vi "lib Read Only 699 Config File.vi"(7 "Mission":string, 8 "error in (no error)":errorcluster, 11 "mission folders in":T1) -> (0 "error out":errorcluster, 3 "mission folders out":T1)   [LabVIEW 2014]
uses:
  lib cluster 699 Config.ctl
  <vilib>/Utility/sysdir.llb/System Directory Type.ctl
  <vilib>/Utility/config.llb/Read Key (String).vi
  <vilib>/Utility/config.llb/NI_LVConfig.lvlib
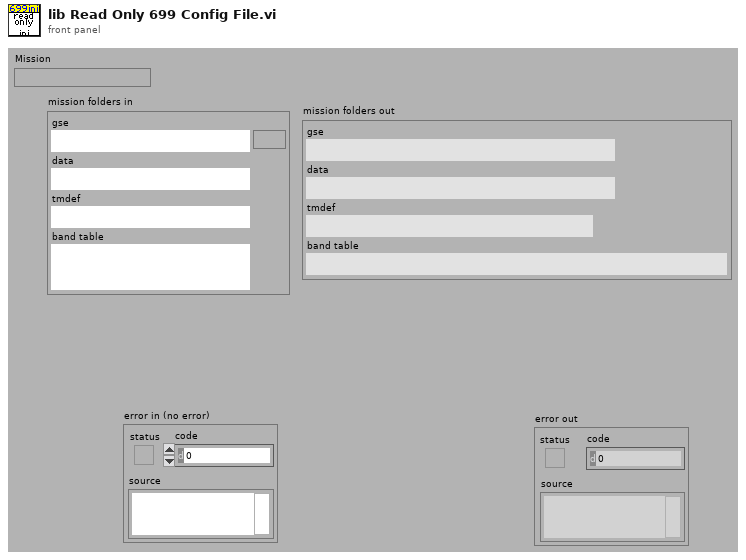
[diagram p1: front panel]
types:
  T1 = typedef "lib cluster 699 Config.ctl" = cluster{"gse":path, "data":path, "tmdef":path, "band table":path}
  T2 = typedef "System Directory Type.ctl" = i32
  T3 = typedef "NI_LVConfig.lvlib/Config Data RefNum.ctl" = refnum<k1>
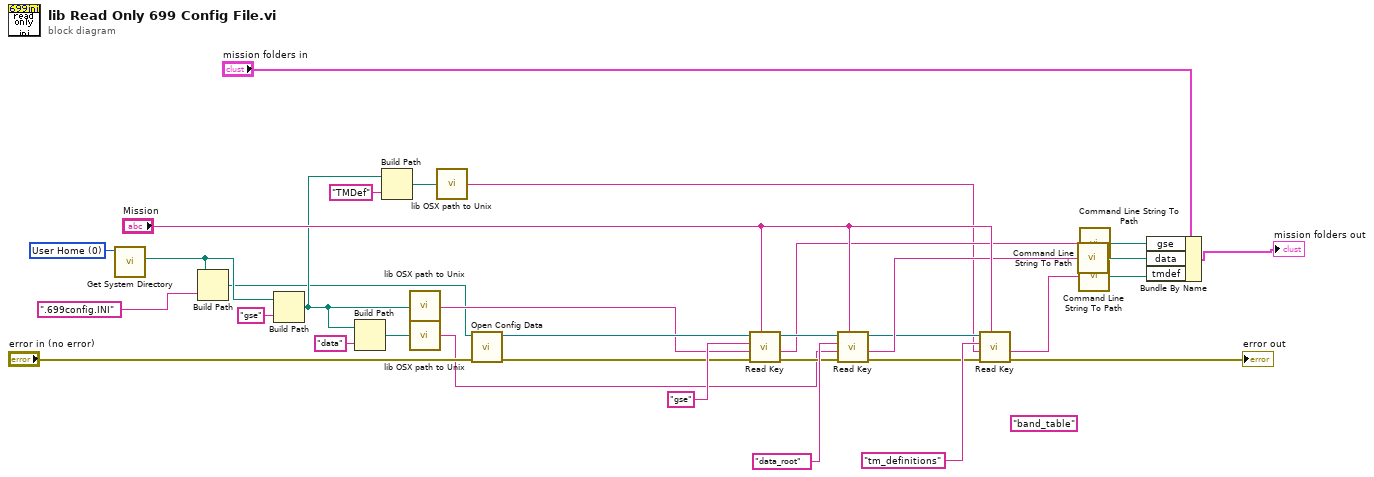
[diagram p0: block diagram]
diagram:
  (unwired) "band_table" ("Item")
  w33 = T2 0 items=["User Home"=0, "User Desktop"=1, "User Documents"=2, "User Application Data"=3, "User Preferences"=4, "User Temporary"=5, "Public Documents"=6, "Public Application Data"=7, "Public Preferences"=8, "Public Cache"=13, "System Core Libraries"=9, "System Installed Libraries"=10, "Application Files"=11, "Boot Volume Root"=12] ("system directory type")
  n1 = call <vilib>:"Get System Directory.vi"("system directory type"=w33) -> ("system directory"=w2:path)  [unwired: 10 in]
  n2 = Build Path(base path=w2, name or relative path=".699config.INI") -> (appended path=w1:path)
  n3 = Build Path(base path=w2, name or relative path="gse") -> (appended path=w20:path)
  n4 = Build Path(base path=w20, name or relative path="data") -> (appended path=w24:path)
  n5 = Build Path(base path=w20, name or relative path="TMDef") -> (appended path=w22:path)
  n6 = call "lib OSX path to Unix.vi"("LV Path"=w20) -> ("UNIX Path"=w11:string)  [unwired: 4 in]
  n7 = call "lib OSX path to Unix.vi"("LV Path"=w24) -> ("UNIX Path"=w8:string)  [unwired: 4 in]
  n8 = call "lib OSX path to Unix.vi"("LV Path"=w22) -> ("UNIX Path"=w5:string)  [unwired: 4 in]
  n9 = call <vilib>:"Open Config Data.vi"("error in (no error)"="error in (no error)", "configuration file path"=w1) -> ("error out"=w13:errorcluster, "refnum"=w12:T3)  [unwired: 7 in, 1 out]
  n10 = call-poly <vilib>:"Read Key.vi"("section"="Mission", "error in (no error)"=w13, "default value"=w11, "key"="gse" ("Item"), "refnum"=w12) -> ("error out"=w19:errorcluster, "value"=w9:string, "refnum out"=w10:T3)  [unwired: 3 in, 1 out]
  n11 = call-poly <vilib>:"Read Key.vi"("section"="Mission", "error in (no error)"=w19, "default value"=w8, "key"="data_root" ("Item"), "refnum"=w10) -> ("error out"=w16:errorcluster, "value"=w7:string, "refnum out"=w6:T3)  [unwired: 3 in, 1 out]
  n12 = call-poly <vilib>:"Read Key.vi"("section"="Mission", "error in (no error)"=w16, "default value"=w5, "key"="tm_definitions" ("Item"), "refnum"=w6) -> ("error out"=→"error out":errorcluster, "value"=w3:string)  [unwired: 3 in, 2 out]
  n13 = call <vilib>:"Command Line String To Path.vi"("string"=w7) -> ("path"=w18:path)
  n14 = call <vilib>:"Command Line String To Path.vi"("string"=w3) -> ("path"=w15:path)
  n15 = call <vilib>:"Command Line String To Path.vi"("string"=w9) -> ("path"=w17:path)
  n16 = Bundle By Name(cluster="mission folders in", "gse"=w17, "data"=w18, "tmdef"=w15) -> (→"mission folders out":T1)
